vi "nonlinearcancellationVolFlow.vi"(10 "input variable":dbl) -> (2 "MVT Process Variable":dbl)   [LabVIEW 2022 SP3]
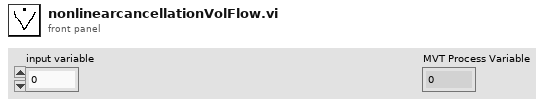
[diagram p1: front panel]
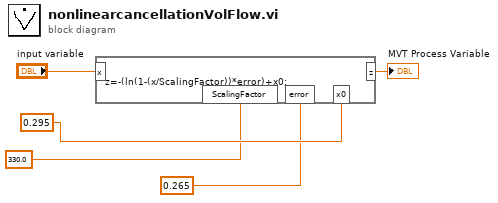
[diagram p0: block diagram]
diagram:
  n1 = formula code="z=-(ln(1-(x/ScalingFactor))*error)+x0;"("x"="input variable", "x0"=0.295, "ScalingFactor"=330.0, "error"=0.265) -> ("z"=→"MVT Process Variable":dbl)
